vi "UnReserveDependency.vi"(7 "Reserving Entity":refnum<class "SMO.lvclass">, 8 "error in (no error)":errorcluster, 9 "Lock Key (if no reserving entity)":string caption="LockKey", 11 "SMO":refnum<class "SMO.lvclass">) -> (0 "error out":errorcluster, 1 "unreserved":bool, 3 "SMO out":refnum<class "SMO.lvclass">)   [LabVIEW 2013, in "SMO.lvclass"]
doc: "SMO terminal to be connected with the resource that is to be unreserved.\nReserving Entity is to be the reference to the object that unreserves the SMO."
uses:
  SMO.lvclass
  SMO.lvclass/SMO.ctl
  Typedefs/Reserve State--Enum.ctl
  Support/Attribute.Owner/Attribute.Owner.lvclass
panel:
  # "For instructions on how to use the JKI State Machine Objects, examples and video tutorials, visit:\nhttp://jki.net/state-machine-objects/\n\nJKI State Machine Objects™\nhttp://jki.net/state-machine-objects/\nCopyright (C) 2005-2015, JKI <info@jki.net>\nALL RIGHTS RESERVED"
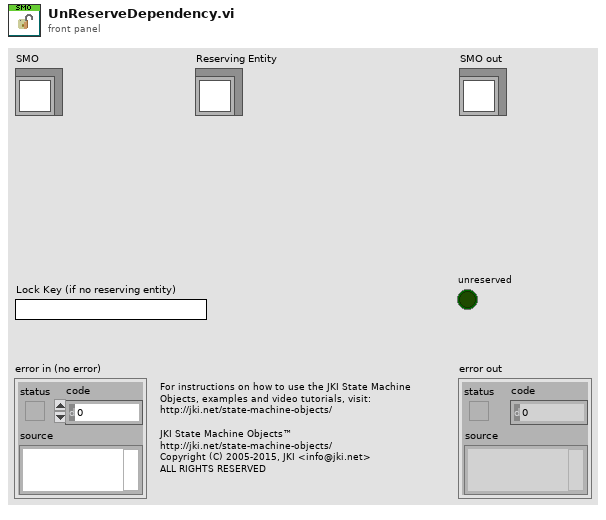
[diagram p1: front panel]
types:
  T1 = typedef "SMO.lvclass/Reserve State--Enum.ctl" = enum16{"Unreserved", "Reserved", "Self-locked"}
  T2 = typedef "SMO.lvclass/PrivateData--Ref.ctl" = refnum<data-value>
  T3 = typedef "SMO.lvclass/PrivateData--Cluster.ctl" = cluster{"Parent Call":T4, "Registered Processes":T5[], "Sync Notifier":refnum<notifier>, "Process Error Notifier":refnum<notifier>, "Protected Events":T6, "Public Events":T7, "SMO State":T8, "[Dependencies]":T9[], "[Attributes]":refnum<class "Attribute.lvclass">[], "Launcher Close":refnum<notifier>, "Caller Watchdog":refnum<queue>, "Accessibility":T10}
  T4 = typedef "SMO.lvclass/Parent Call--Enum.ctl" = enum16{"Allows parent to run", "Does not request parent to run"}
  T5 = typedef "SMO.lvclass/RegisteredProcessData--Cluster.ctl" = cluster{"Name":string, "Static VI Ref":refnum<vi>, "Running":bool, "NotifierRef":u32}
  T6 = typedef "SMO.lvclass/Protected Events.ctl" = cluster{"StopProcesses":refnum<user-event>, "AbortProcesses":refnum<user-event>, "Config Changed":refnum<user-event>, "Dependency":refnum<user-event>}
  T7 = typedef "SMO.lvclass/Public Events.ctl" = cluster{"Error":refnum<user-event>, "State":refnum<user-event>, "Reserve State":refnum<user-event>}
  T8 = typedef "SMO.lvclass/SMOState --Enum.ctl" = enum16{"unknown", "Created", "Started", "Stopped"}
  T9 = typedef "SMO.lvclass/SMO Dependency--Cluster.ctl" = cluster{"Dependency":refnum<class "SMO.lvclass">, "Level":string}
  T10 = typedef "SMO.lvclass/Accessibility--Cluster.ctl" = cluster{"Lock Key":string, "Reserve State":T1}
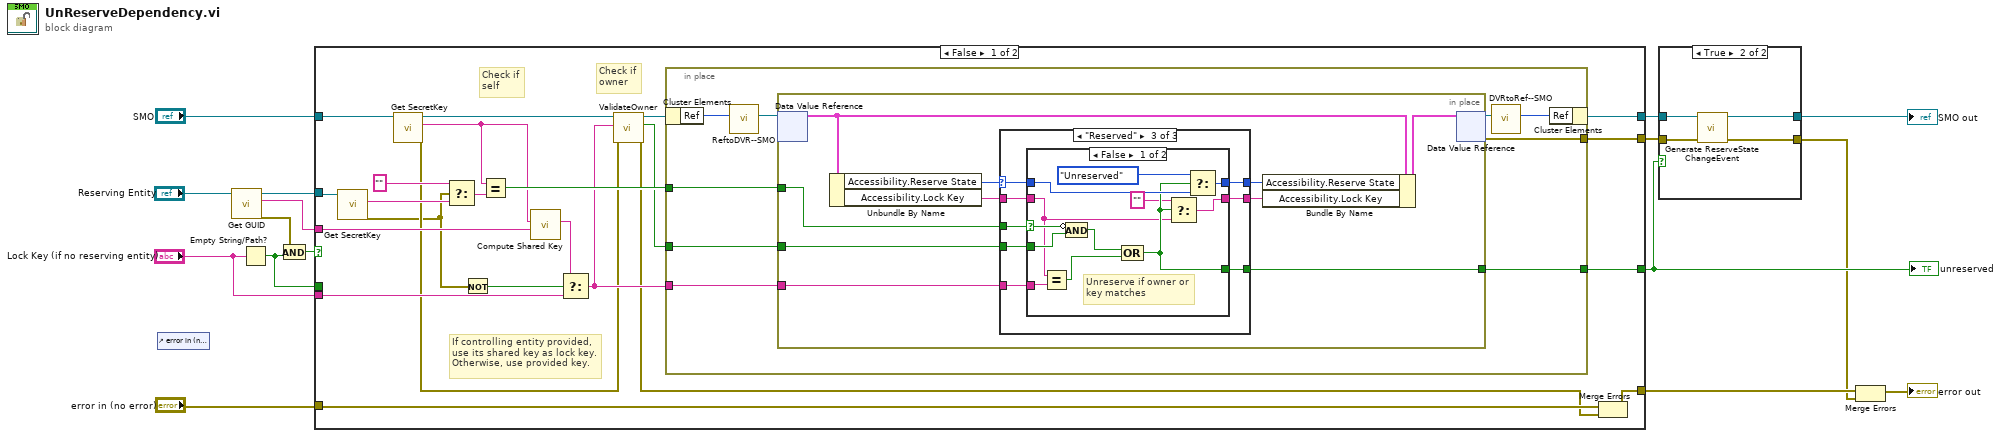
[diagram p0: block diagram]
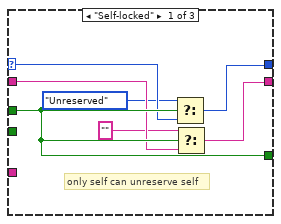
[diagram p3: hidden frame]
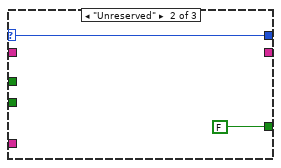
[diagram p4: hidden frame]
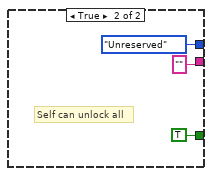
[diagram p5: hidden frame]
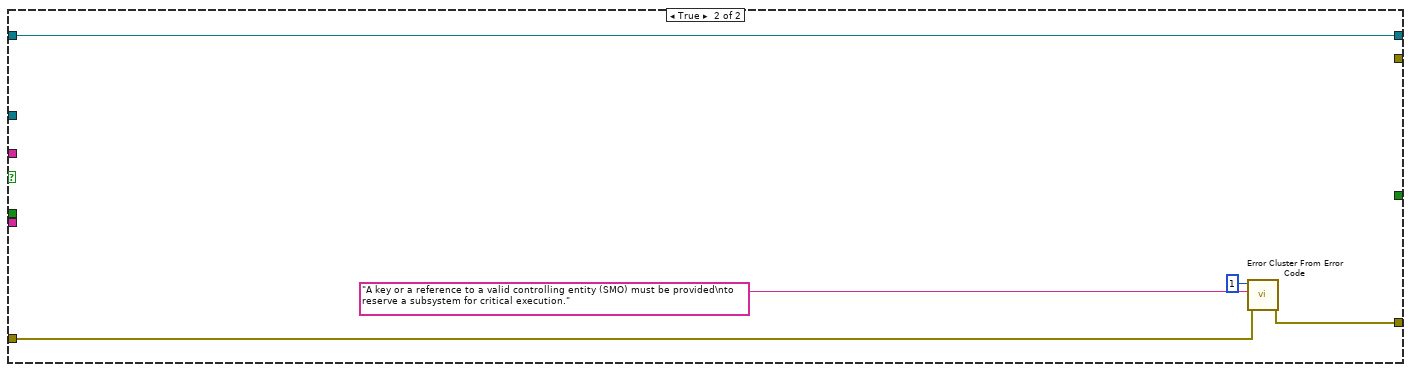
[diagram p6: hidden frame]
diagram:
  n1 = control-ref of="error in (no error)"() -> ()  [unwired: 1 out]
  n2 = call "Get GUID.vi"("SMO"="Reserving Entity") -> ("error out"=w10:errorcluster, "GUID"=w7:string, "SMO out"=w5:refnum<class "SMO.lvclass">)  [unwired: 8 in]
  n3 = Empty String/Path?(string/path="Lock Key (if no reserving entity)") -> (empty?=w6:bool)
  n4 = Compound Arithmetic op=AND(w10, w6) -> (w9:bool)
  n5 = case shown="False" w9 {
    tunnel: [w39 w95] -> w4
    tunnel: [w38 _] -> w3
    tunnel: "SMO" -> [w28 w95]
    tunnel: [w17 w94] -> w8
    tunnel: "error in (no error)" -> [w19 w91]
    tunnel: w7 -> [w37 _]
    tunnel: "Lock Key (if no reserving entity)" -> [w35 _]
    tunnel: w6 -> [_ _]
    tunnel: w5 -> [w34 _]
    tunnel: [w20 _] -> w11
    frame False {
      # "If controlling entity provided,\nuse its shared key as lock key.\nOtherwise, use provided key."
      # "Check if\nself"
      # "Check if\nowner"
      n6 = call "Get SecretKey.vi"("SMO"=w34) -> ("error out"=w22:errorcluster, "SecretKey"=w33:string)  [unwired: 8 in, 1 out]
      n7 = call "Get SecretKey.vi"("SMO"=w28) -> ("error out"=w24:errorcluster, "SecretKey"=w29:string, "SMO out"=w27:refnum<class "SMO.lvclass">)  [unwired: 8 in]
      n8 = Select(t="", s=w22, f=w33) -> (s? t:f=w31:string)
      n9 = Not(x=w22) -> (.not. x?=w21:bool)
      n10 = Equal?(x=w29, y=w31) -> (x = y?=w30:bool)
      n11 = call "Compute Shared Key.vi"("GUID"=w37, "SecretKey"=w29) -> ("Shared Key"=w36:string)  [unwired: 9 in]
      n12 = Select(t=w36, s=w21, f=w35) -> (s? t:f=w25:string)
      n13 = call "ValidateOwner.vi"("error in (no error)"=w24, "Shared Key"=w25, "SMO in"=w27) -> ("error out"=w18:errorcluster, "key matched"=w23:bool, "SMO out"=w26:refnum<class "SMO.lvclass">)  [unwired: 6 in]
      n14 = in-place {
        in-place-border: [w48] -> w38
        in-place-border: w25 -> [w43]
        in-place-border: w30 -> [w42]
        in-place-border: w23 -> [w41]
        in-place-border: [w40] -> w20
        n15 = in-place-cluster #1(w26) -> ("Ref"=w47:u32)
        n16 = call "ReftoDVR--SMO.vi"("Ref"=w47) -> ("Ref"=w46:T2)  [unwired: 10 in]
        n17 = in-place {
          in-place-border: w43 -> [w55]
          in-place-border: w42 -> [w52]
          in-place-border: w41 -> [w50]
          in-place-border: [w49] -> w40
          n18 = in-place-dvr #2(w46) -> (w57:T3)  [unwired: 1 out]
          n19 = Unbundle By Name(w57) -> ("Accessibility.Reserve State"=w58:T1, "Accessibility.Lock Key"=w51:string)
          n20 = case shown="\"Reserved\"" w58 {
            selector: w58 -> [w64 w67 w71]
            tunnel: w55 -> [_ _ w72]
            tunnel: [w61 _ w73] -> w54
            tunnel: [w63 w67 w74] -> w53
            tunnel: w52 -> [w65 _ w75]
            tunnel: w51 -> [w62 _ w70]
            tunnel: w50 -> [_ _ w69]
            tunnel: [w65 FALSE w68] -> w49
            frame "Self-locked" {
              # "only self can unreserve self"
              n21 = Select(t=Reserve_State--Enum."Unreserved", s=w65, f=w64) -> (s? t:f=w63:T1)
              n22 = Select(t="", s=w65, f=w62) -> (s? t:f=w61:string)
            }
            frame "Unreserved" {
            }
            frame "Reserved" {
              n23 = case shown="False" w75 {
                selector: w75 -> [w87 _]
                tunnel: [w83 Reserve_State--Enum."Unreserved" ("Reserve State")] -> w74
                tunnel: [w78 "" ("Lock Key")] -> w73
                tunnel: w72 -> [w81 _]
                tunnel: w71 -> [w85 _]
                tunnel: w70 -> [w77 _]
                tunnel: w69 -> [w86 _]
                tunnel: [w79 TRUE] -> w68
                frame False {
                  # "Unreserve if owner or\nkey matches"
                  n24 = Equal?(x=w77, y=w81) -> (x = y?=w80:bool)
                  n25 = Compound Arithmetic op=AND(invert w87, w86) -> (w82:bool)
                  n26 = Compound Arithmetic op=OR(w82, w80) -> (w79:bool)
                  n27 = Select(t="", s=w79, f=w77) -> (s? t:f=w78:string)
                  n28 = Select(t=Reserve_State--Enum."Unreserved" ("Accessibility.Reserve State"), s=w79, f=w85) -> (s? t:f=w83:T1)
                }
                frame True {
                  # "Self can unlock all"
                }
              }
            }
          }
          n29 = Bundle By Name(cluster=w57, "Accessibility.Reserve State"=w53, "Accessibility.Lock Key"=w54) -> (w56:T3)
          n30 = in-place-dvr #2(w56) -> (w45:T2, w48:errorcluster)
        }
        n31 = call "DVRtoRef--SMO.vi"("Ref"=w45) -> ("Ref"=w44:u32)  [unwired: 10 in]
        n32 = in-place-cluster #1("Ref"=w44) -> (w39:refnum<class "SMO.lvclass">)
      }
      n33 = Merge Errors(w19, w18) -> (w17:errorcluster)
    }
    frame True {
      n34 = call <vilib>:"Error Cluster From Error Code.vi"("error in (no error)"=w91, "error message (\"\")"="A key or a reference to a valid controlling entity (SMO) must be provided\nto reserve a subsystem for critical execution." ("error message (\"\")"), "error code (0)"=1) -> ("error out"=w94:errorcluster)  [unwired: 6 in]
    }
  }
  "unreserved" <- w11
  n35 = case shown="True" w11 {
    tunnel: w4 -> [w97 w101]
    tunnel: [w97 w99] -> w1
    tunnel: [w96 w98] -> w2
    tunnel: w3 -> [w96 w100]
    frame False {
    }
    frame True {
      n36 = call "Generate ReserveState ChangeEvent.vi"("error in (no error)"=w100, "SMO in"=w101) -> ("error out"=w98:errorcluster, "SMO out"=w99:refnum<class "SMO.lvclass">)  [unwired: 8 in]
    }
  }
  "SMO out" <- w1
  n37 = Merge Errors(w8, w2) -> (→"error out":errorcluster)
